vi "Query Trigger Connector Catalog With Format.vi"(8 "error in (no error)":errorcluster, 10 "Format (Default)":i32(ring) items=["Default", "Fully Qualified Name", "Label Only"], 11 "VISA resource name":refnum<visa-resource-name>) -> (0 "error out":errorcluster, 2 "Connectors":string, 3 "VISA resource name out":refnum<visa-resource-name>)   [LabVIEW 2020, in "Rohde&Schwarz CMXP Base.lvlib"]
doc: "Lists all trigger connectors of the primary instrument and of all instruments controlled by the primary instrument. Allows user to select the response format.\n\nAttribute:\nRSCMXPBASE_ATTR_TRIGGER_CONNECTOR_CATALOG\n\nRemote-control command:\nTRIGger:BASE:EXTernal:CATalog?"
uses:
  <instrlib>/Rohde&Schwarz CMXP Base/Rohde&Schwarz CMXP Base.lvlib
  <instrlib>/Rohde&Schwarz CMXP Base/Private/rsidr_core.llb/rsidr_core.lvlib
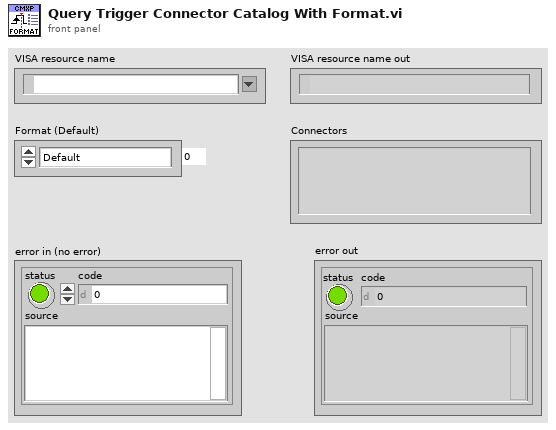
[diagram p1: front panel]
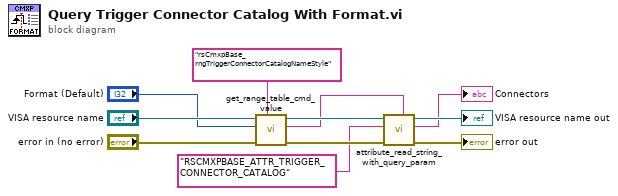
[diagram p0: block diagram]
diagram:
  n1 = call <instrlib>:"get_range_table_cmd_value.vi"("Range Table ID in"="rsCmxpBase_rngTriggerConnectorCatalogNameStyle", "error in"="error in (no error)", "Input Int32 value"="Format (Default)", "VISA resource name"="VISA resource name") -> ("error out"=w8:errorcluster, "Cmd value out"=w6:string, "VISA resource name out"=w9:refnum<visa-resource-name>)  [unwired: 5 in]
  n2 = call <instrlib>:"attribute_read_string_with_query_param.vi"("Query Parameter (None)"=w6, "error in"=w8, "Attribute ID"="RSCMXPBASE_ATTR_TRIGGER_CONNECTOR_CATALOG", "VISA resource name"=w9) -> ("error out"=→"error out":errorcluster, "String out"=→"Connectors":string, "VISA resource name out"=→"VISA resource name out":refnum<visa-resource-name>)  [unwired: 5 in]
